vi "Goalie.vi"(9 "IA Input":T3, 10 "Robot":T1, 11 "command\nenum":T7) -> (2 "output cluster":T1)   [LabVIEW 2016]
uses:
  Core/AI Robot.ctl
  Functions Enum.ctl
  Command Enum.ctl
  Core/AI Input.ctl
  Core/AI Ball.ctl
  Core/Field Size.ctl
  Core/AI Judge.ctl
  <vilib>/Analysis/_algsub.llb/Real Vector Norm.vi
  <vilib>/Analysis/NI_AALPro.lvlib
panel:
  in  "min dist to kick 2":dbl=195.0 format="%#_13g"
  in  "attck contra?":dbl
  in  "min dist to kick":dbl=195.0 format="%#_13g"
  in  "T":dbl[](array[numeric])
  in  "Vel min":dbl=10.0 format="%#_13g"
  in  "Attacker Distance":dbl=200.0
  out "Closest Robot":T1
  out "Max Dist":dbl=999999999.0 format="%#_13g"
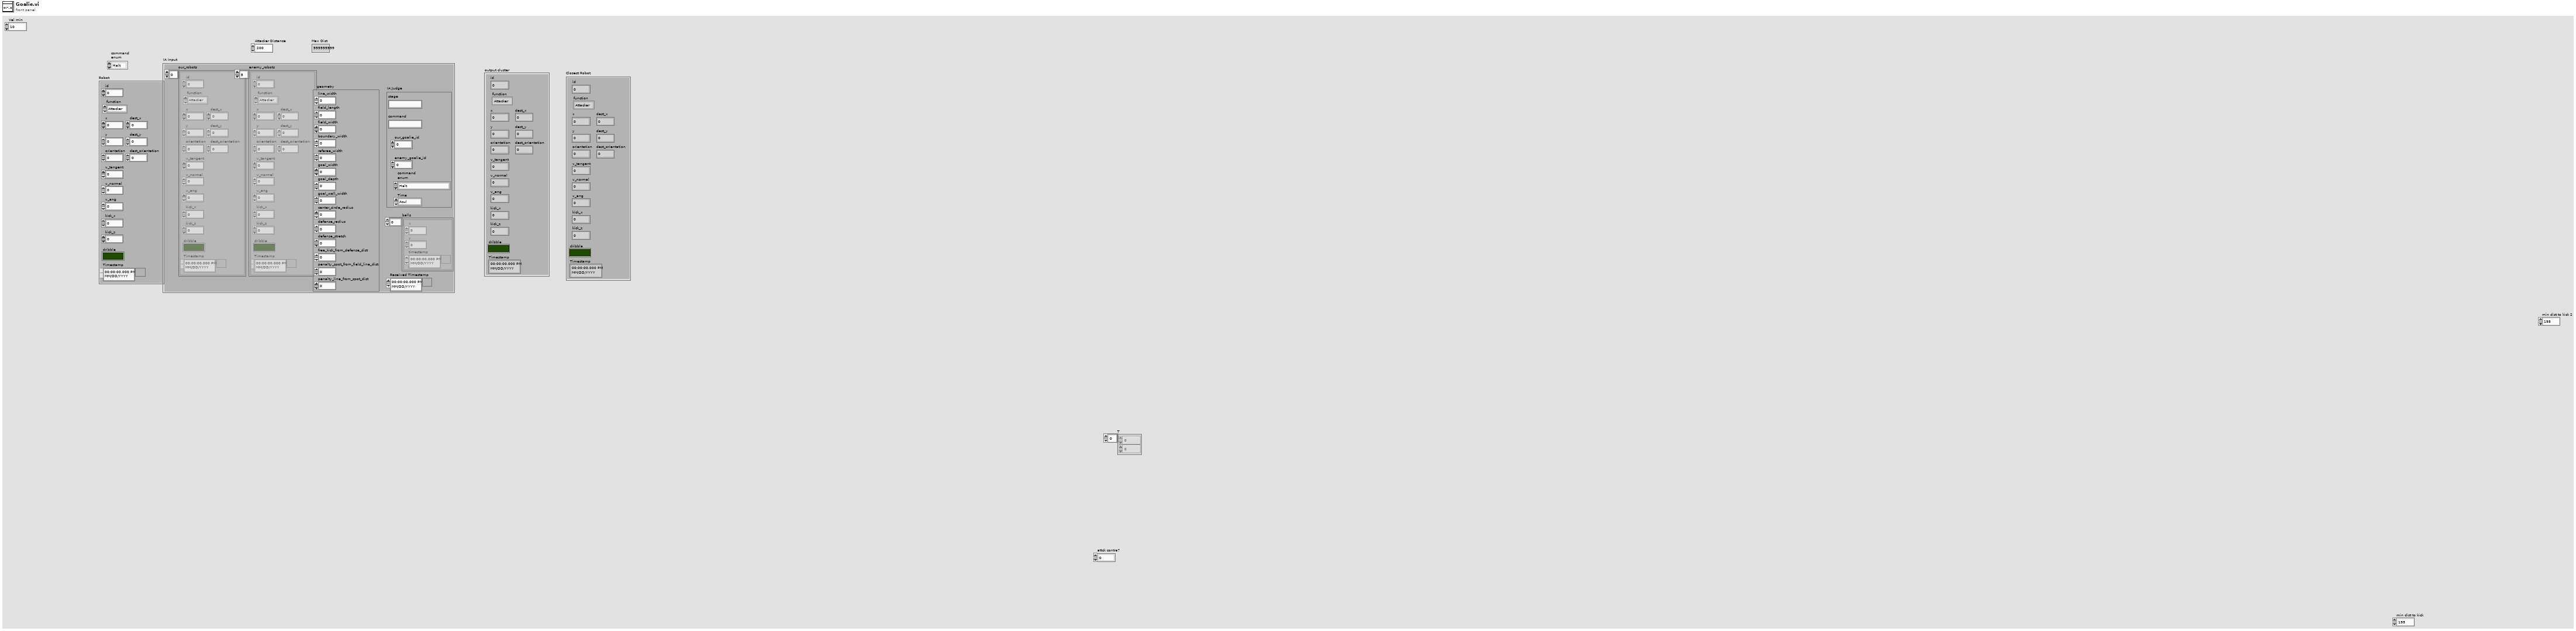
[diagram p1: front panel]
types:
  T1 = typedef "AI Robot.ctl" = cluster{"id":u32, "function":T2, "x":dbl, "y":dbl, "orientation":dbl, "v_tangent":dbl, "v_normal":dbl, "v_ang":dbl, "kick_x":dbl, "kick_z":dbl, "dribble":bool, "Timestamp":timestamp, "dest_x":dbl, "dest_y":dbl, "dest_orientation":dbl}
  T2 = typedef "Functions Enum.ctl" = enum16{"Attacker", "Goalie", "Defender", "Goto 0", "Dummy", "ZigZag"}
  T3 = typedef "AI Input.ctl" = cluster{"our_robots":T1[], "enemy_robots":T1[], "balls":T4[], "geometry":T5, "IA Judge":T6, "Received Timestamp":timestamp}
  T4 = typedef "AI Ball.ctl" = cluster{"x":dbl, "y":dbl, "timestamp":timestamp}
  T5 = typedef "Field Size.ctl" = cluster{"line_width":u32, "field_length":u32, "field_width":u32, "boundary_width":u32, "referee_width":u32, "goal_width":u32, "goal_depth":u32, "goal_wall_width":u32, "center_circle_radius":u32, "defense_radius":u32, "defense_stretch":u32, "free_kick_from_defense_dist":u32, "penalty_spot_from_field_line_dist":u32, "penalty_line_from_spot_dist":u32}
  T6 = typedef "AI Judge.ctl" = cluster{"stage":string, "command":string, "our_goalie_id":dbl, "enemy_goalie_id":dbl, "command\nenum":T7, "Time":enum16{"Azul", "Amarelo"}}
  T7 = typedef "Command Enum.ctl" = enum16{"Halt", "Stop", "Force Start", "PKA Normal Start", "Prepare Kickoff Ally", "PKE Normal Start", "Prepare Kickoff Enemy", "Prepare Penalty Ally", "PPA Normal Start", "Prepare Penalty Enemy", "PPE Normal Start", "Direct Free Enemy", "Direct Free Ally", "Indirect Free Enemy", "Indirect Free Ally", "Timeout Enemy", "Timeout Ally", "Goal Enemy", "Goal Ally", "Ball Placement Enemy", "Ball Placement Ally", "None"}
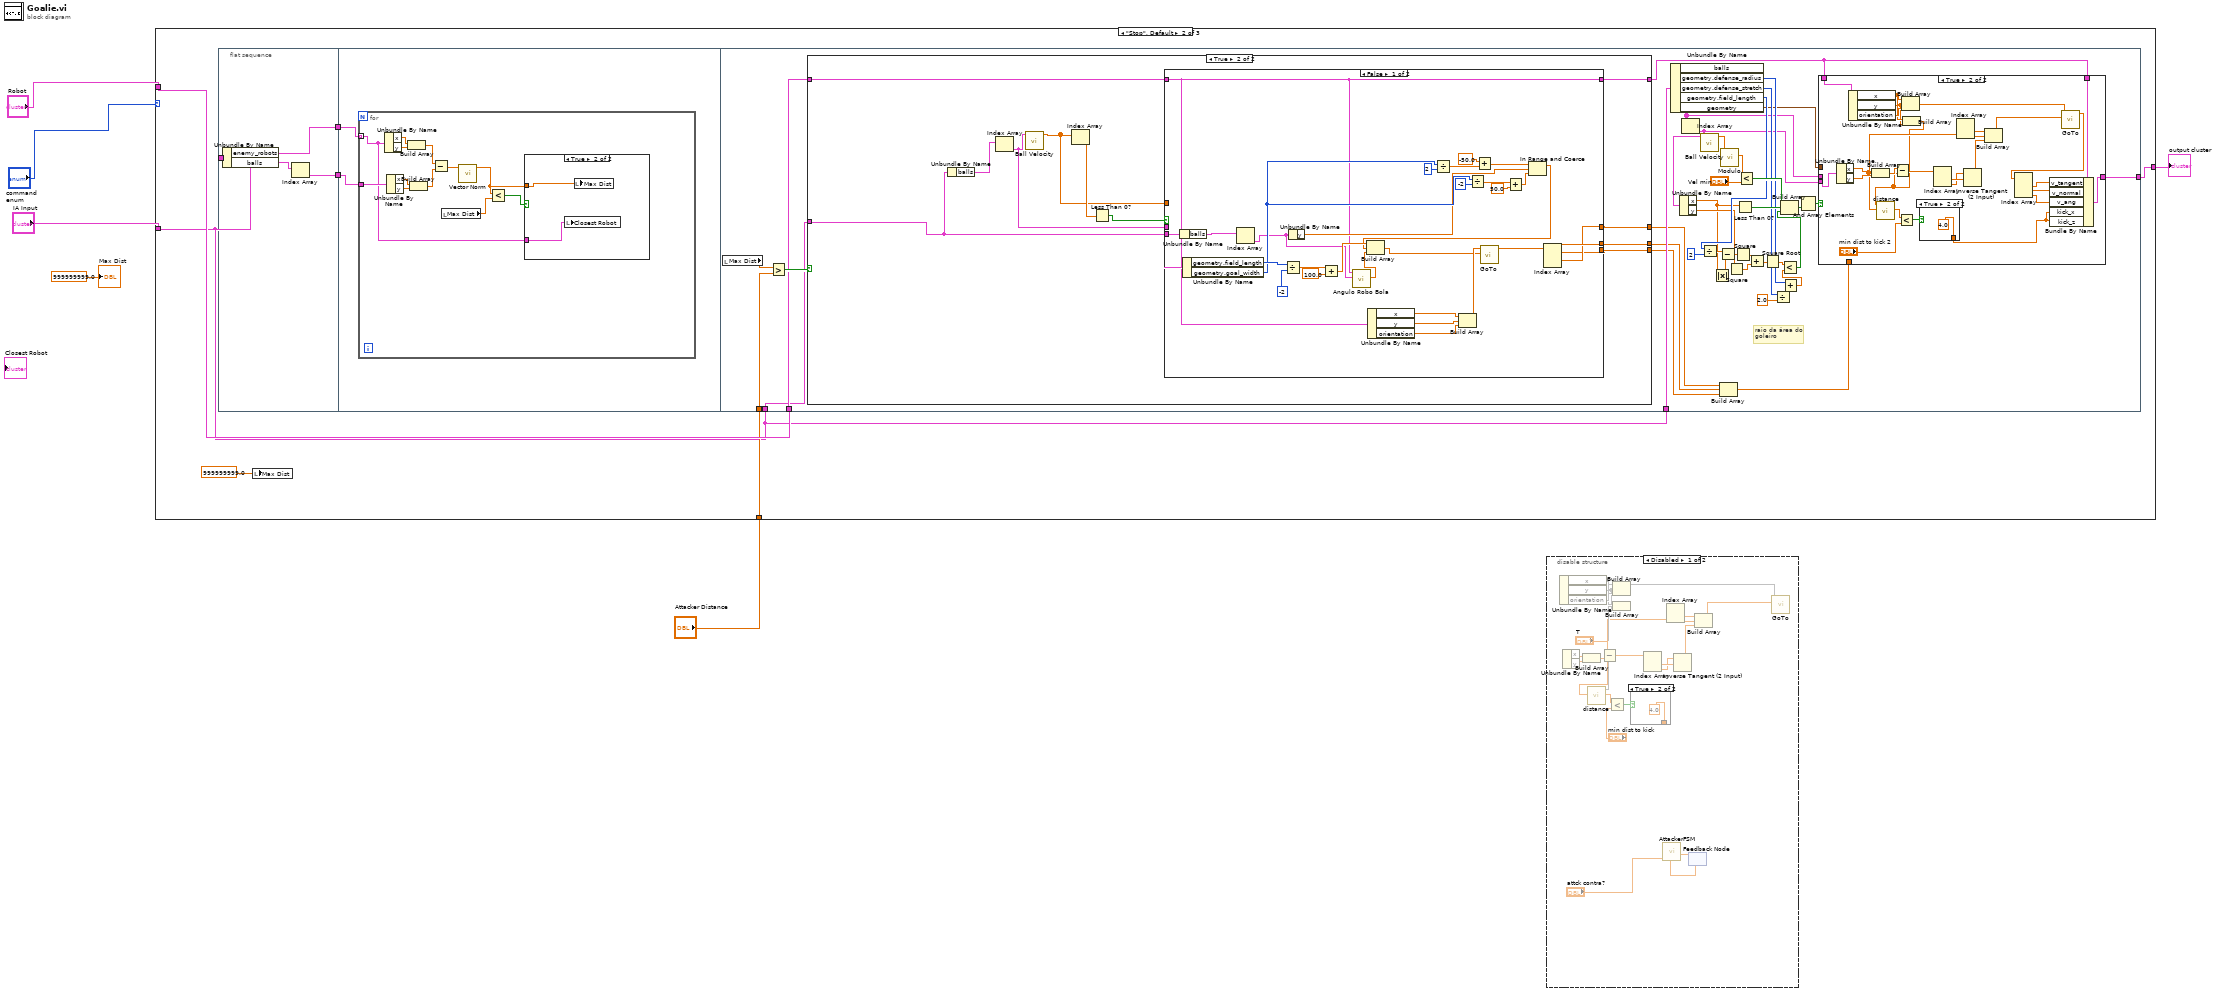
[diagram p0: block diagram]
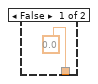
[diagram p2: hidden frame]
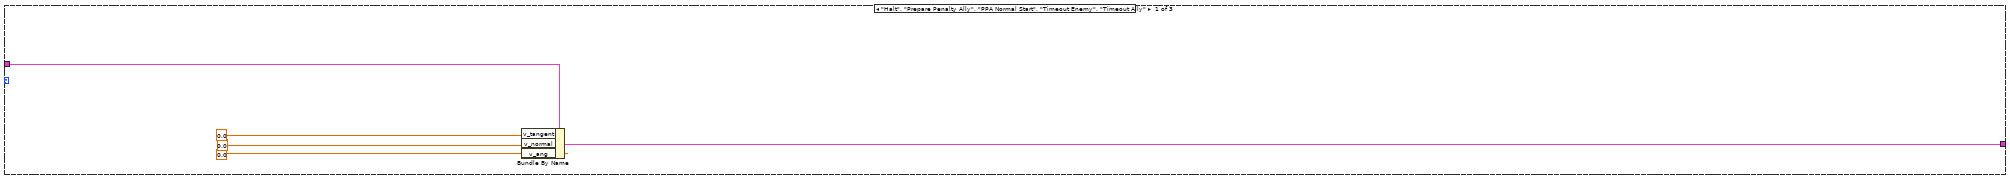
[diagram p4: hidden frame]
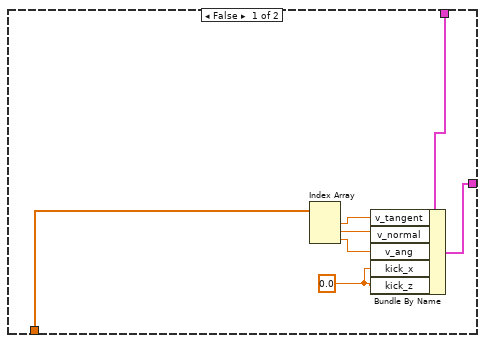
[diagram p6: hidden frame]
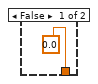
[diagram p7: hidden frame]
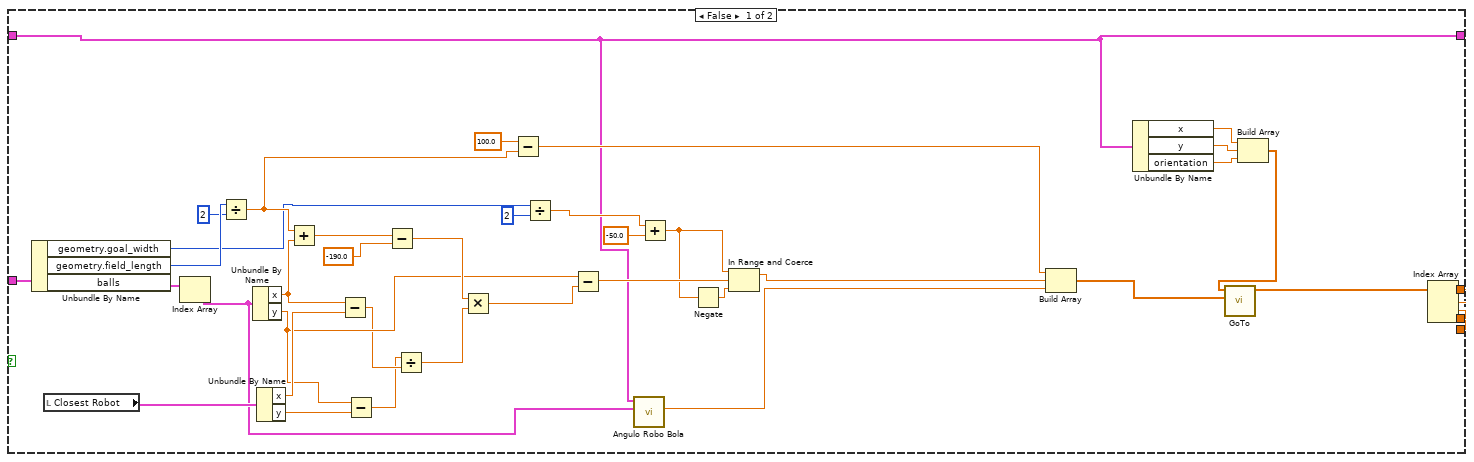
[diagram p8: hidden frame]
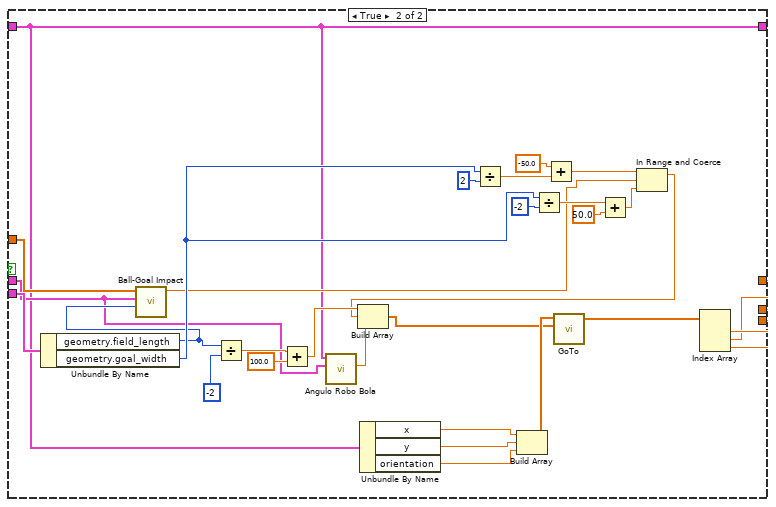
[diagram p9: hidden frame]
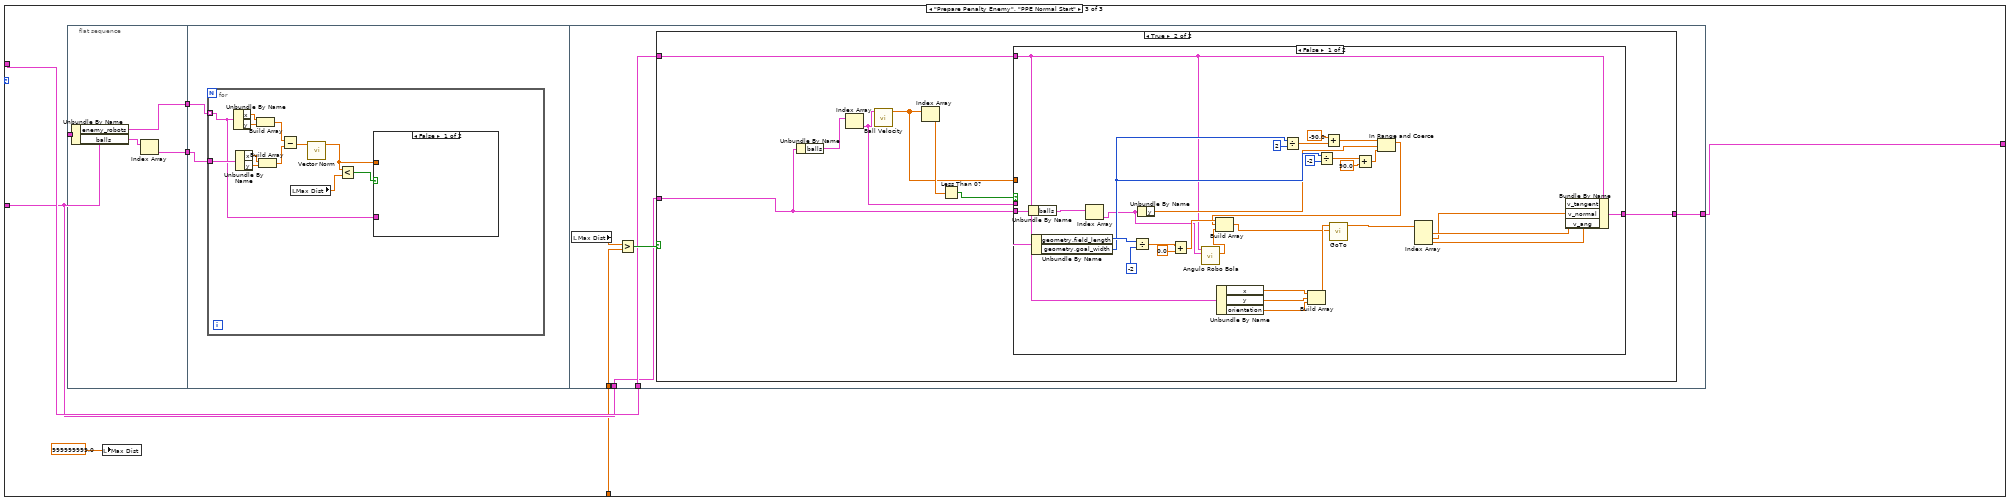
[diagram p10: hidden frame]
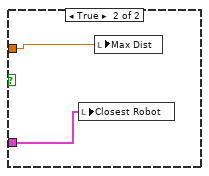
[diagram p11: hidden frame]
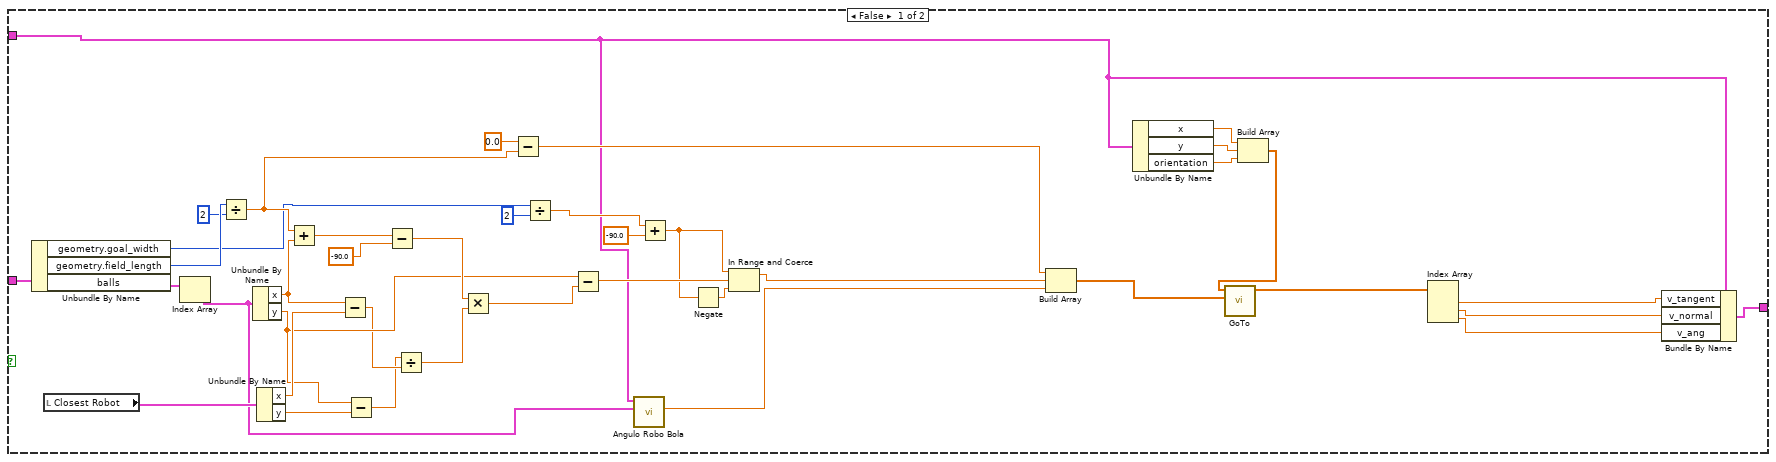
[diagram p12: hidden frame]
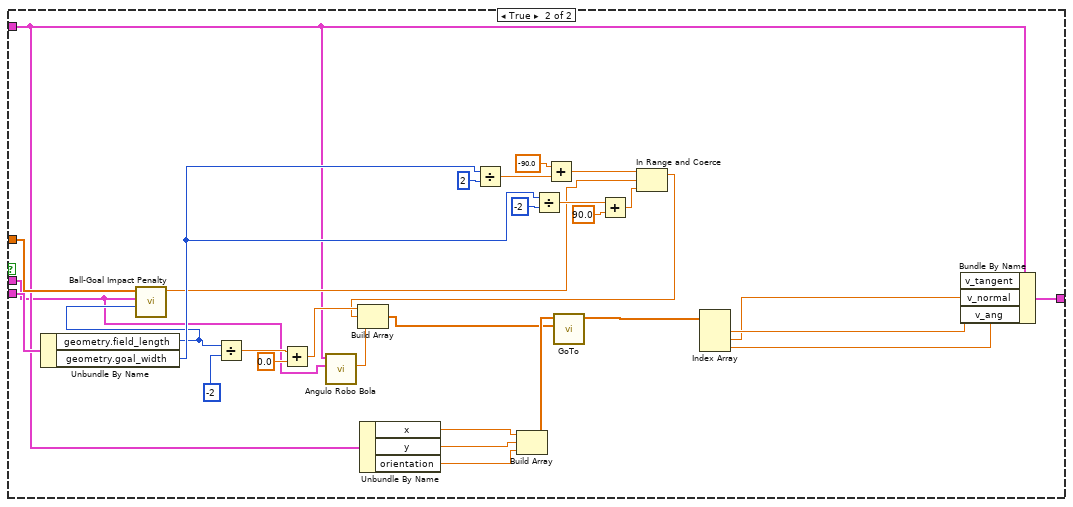
[diagram p13: hidden frame]
diagram:
  n1 = case shown="\"Stop\", Default" "command\nenum" {
    tunnel: "Robot" -> [w11 w16 w228]
    tunnel: [w7 w12 w226] -> w3
    tunnel: "IA Input" -> [_ w13 w227]
    tunnel: "Attacker Distance" -> [_ w15 w225]
    frame "Halt", "Prepare Penalty Ally", "PPA Normal Start", "Timeout Enemy", "Timeout Ally" {
      n2 = Bundle By Name(cluster=w11, "v_tangent"=0.0 ("v_x"), "v_normal"=0.0 ("v_y"), "v_ang"=0.0) -> (w7:T1)
    }
    frame "Stop", Default {
      n3 = flat-sequence {
        tunnel: w13 -> [w22]
        tunnel: [w21] -> w18
        tunnel: [w19] -> w17
        tunnel: w18 -> [w24]
        tunnel: w17 -> [w23]
        tunnel: w16 -> [w75]
        tunnel: w13 -> [w74]
        tunnel: w15 -> [w73]
        tunnel: w13 -> [w72]
        tunnel: [w41] -> w12
        frame #0 {
          n4 = Unbundle By Name(w22) -> ("enemy_robots"=w21:T1[], "balls"=w20:T4[])
          n5 = Index Array(array=w20) -> (element=w19:T4)  [unwired: 1 in]
        }
        frame #1 {
          n6 = for {
            tunnel: w24 -> [w26] mode=indexing
            tunnel: w23 -> [w36]
            n7 = Unbundle By Name(w26) -> ("x"=w35:dbl, "y"=w34:dbl)
            n8 = Unbundle By Name(w36) -> ("x"=w33:dbl, "y"=w32:dbl)
            n9 = Build Array(w35, w34) -> (w31:dbl[])
            n10 = Build Array(w33, w32) -> (w30:dbl[])
            n11 = Subtract(x=w31, y=w30) -> (x-y=w29:dbl[])
            n12 = local read "Max Dist"() -> (w28:dbl)
            n13 = call-poly <vilib>:"Vector Norm.vi"("Input Vector"=w29) -> ("norm"=w25:dbl)  [unwired: 9 in, 1 out]
            n14 = Less?(x=w25, y=w28) -> (x < y?=w27:bool)
            n15 = case shown="True" w27 {
              tunnel: w26 -> [_ w38]
              tunnel: w25 -> [_ w37]
              frame False {
              }
              frame True {
                n16 = local write "Closest Robot"(w38) -> ()
                n17 = local write "Max Dist"(w37) -> ()
              }
            }
          }
        }
        frame #2 {
          # "raio da área do \ngoleiro"
          n18 = local read "Max Dist"() -> (w76:dbl)
          n19 = Greater?(x=w76, y=w73) -> (0:w77:bool)
          n20 = case shown="True" w77 {
            tunnel: w75 -> [w114 w163]
            tunnel: w74 -> [w152 w162]
            tunnel: [w117 w156] -> w68
            tunnel: [w116 w155] -> w66
            tunnel: [w115 w154] -> w69
            tunnel: [w114 w153] -> w40
            frame False {
              n21 = Unbundle By Name(w152) -> ("geometry.goal_width"=w126:u32, "geometry.field_length"=w148:u32, "balls"=w151:T4[])
              n22 = local read "Closest Robot"() -> (w150:T1)
              n23 = Index Array(array=w151) -> (element=w119:T4)  [unwired: 1 in]
              n24 = Divide(x=w148, y=u32 2) -> (x/y=w137:dbl)
              n25 = Unbundle By Name(w119) -> ("x"=w146:dbl, "y"=w140:dbl)
              n26 = Unbundle By Name(w150) -> ("x"=w149:dbl, "y"=w139:dbl)
              n27 = Add(x=w137, y=w146) -> (x+y=w145:dbl)
              n28 = Subtract(x=w146, y=w149) -> (x-y=w129:dbl)
              n29 = Subtract(x=w140, y=w139) -> (x-y=w128:dbl)
              n30 = Subtract(x=w145, y=-190.0) -> (x-y=w143:dbl)
              n31 = Divide(x=w128, y=w129) -> (x/y=w142:dbl)
              n32 = Multiply(x=w143, y=w142) -> (x*y=w141:dbl)
              n33 = Subtract(x=100.0, y=w137) -> (x-y=w136:dbl)
              n34 = Divide(x=w126, y=u32 2) -> (x/y=w124:dbl)
              n35 = Subtract(x=w140, y=w141) -> (x-y=w127:dbl)
              n36 = call "Angulo Robo Bola.vi"("Ball"=w119, "Robot"=w114) -> ("Angulo"=w118:dbl)  [unwired: 9 in]
              n37 = Add(x=w124, y=-50.0) -> (x+y=w121:dbl)
              n38 = Negate(x=w121) -> (-x=w122:dbl)
              n39 = In Range and Coerce(upper limit=w121, x=w127, lower limit=w122) -> (coerced(x)=w120:dbl)  [unwired: 1 out]
              n40 = Build Array(w136, w120, w118) -> (w135:dbl[])
              n41 = Unbundle By Name(w114) -> ("x"=w134:dbl, "y"=w133:dbl, "orientation"=w132:dbl)
              n42 = Build Array(w134, w133, w132) -> (w131:dbl[])
              n43 = call "GoTo.vi"("Target"=w135, "Position"=w131) -> ("Output\nVelocity"=w130:dbl[])  [unwired: 8 in, 1 out]
              n44 = Index Array(array=w130) -> (element #1=w117:dbl, element #2=w116:dbl, element #3=w115:dbl)  [unwired: 3 in]
            }
            frame True {
              n45 = Unbundle By Name(w162) -> ("balls"=w161:T4[])
              n46 = Index Array(array=w161) -> (element=w157:T4)  [unwired: 1 in]
              n47 = call "Ball Velocity.vi"("Ball"=w157) -> ("Velocity"=w158:dbl[])  [unwired: 10 in]
              n48 = Index Array(array=w158) -> (element=w160:dbl)  [unwired: 1 in]
              n49 = Less Than 0?(x=w160) -> (x < 0?=w159:bool)
              n50 = case shown="False" w159 {
                tunnel: w162 -> [w189 w219]
                tunnel: w163 -> [w167 w194]
                tunnel: w158 -> [_ w201]
                tunnel: w157 -> [_ w199]
                tunnel: [w166 w197] -> w156
                tunnel: [w165 w196] -> w155
                tunnel: [w164 w195] -> w154
                tunnel: [w167 w194] -> w153
                frame False {
                  n51 = Unbundle By Name(w189) -> ("balls"=w188:T4[])
                  n52 = Unbundle By Name(w189) -> ("geometry.field_length"=w187:u32, "geometry.goal_width"=w180:u32)
                  n53 = Index Array(array=w188) -> (element=w169:T4)  [unwired: 1 in]
                  n54 = Divide(x=w187, y=-2) -> (x/y=w186:dbl)
                  n55 = Unbundle By Name(w169) -> ("y"=w176:dbl)
                  n56 = Add(x=w186, y=100.0) -> (x+y=w184:dbl)
                  n57 = call "Angulo Robo Bola.vi"("Ball"=w169, "Robot"=w167) -> ("Angulo"=w168:dbl)  [unwired: 9 in]
                  n58 = Unbundle By Name(w167) -> ("x"=w191:dbl, "y"=w193:dbl, "orientation"=w192:dbl)
                  n59 = Divide(x=w180, y=2) -> (x/y=w173:dbl)
                  n60 = Build Array(w191, w193, w192) -> (w183:dbl[])
                  n61 = Divide(x=w180, y=-2) -> (x/y=w175:dbl)
                  n62 = Add(x=-50.0, y=w173) -> (x+y=w171:dbl)
                  n63 = Add(x=w175, y=50.0) -> (x+y=w170:dbl)
                  n64 = In Range and Coerce(upper limit=w171, x=w176, lower limit=w170) -> (coerced(x)=w177:dbl)  [unwired: 1 out]
                  n65 = Build Array(w184, w177, w168) -> (w182:dbl[])
                  n66 = call "GoTo.vi"("Target"=w182, "Position"=w183) -> ("Output\nVelocity"=w181:dbl[])  [unwired: 8 in, 1 out]
                  n67 = Index Array(array=w181) -> (element #1=w166:dbl, element #2=w165:dbl, element #3=w164:dbl)  [unwired: 3 in]
                }
                frame True {
                  n68 = Unbundle By Name(w219) -> ("geometry.field_length"=w202:u32, "geometry.goal_width"=w212:u32)
                  n69 = call "Ball-Goal Impact.vi"("Field Length"=w202, "Ball"=w199, "Ball Velocity"=w201) -> ("Y Collision"=w200:dbl)  [unwired: 8 in]
                  n70 = Divide(x=w202, y=-2) -> (x/y=w218:dbl)
                  n71 = Add(x=w218, y=100.0) -> (x+y=w216:dbl)
                  n72 = call "Angulo Robo Bola.vi"("Ball"=w199, "Robot"=w194) -> ("Angulo"=w198:dbl)  [unwired: 9 in]
                  n73 = Unbundle By Name(w194) -> ("x"=w221:dbl, "y"=w223:dbl, "orientation"=w222:dbl)
                  n74 = Divide(x=w212, y=2) -> (x/y=w206:dbl)
                  n75 = Build Array(w221, w223, w222) -> (w215:dbl[])
                  n76 = Divide(x=w212, y=-2) -> (x/y=w208:dbl)
                  n77 = Add(x=-50.0, y=w206) -> (x+y=w204:dbl)
                  n78 = Add(x=w208, y=50.0) -> (x+y=w203:dbl)
                  n79 = In Range and Coerce(upper limit=w204, x=w200, lower limit=w203) -> (coerced(x)=w209:dbl)  [unwired: 1 out]
                  n80 = Build Array(w216, w209, w198) -> (w214:dbl[])
                  n81 = call "GoTo.vi"("Target"=w214, "Position"=w215) -> ("Output\nVelocity"=w213:dbl[])  [unwired: 8 in, 1 out]
                  n82 = Index Array(array=w213) -> (element #1=w197:dbl, element #2=w196:dbl, element #3=w195:dbl)  [unwired: 3 in]
                }
              }
            }
          }
          n83 = Unbundle By Name(w72) -> ("balls"=w43:T4[], "geometry.defense_radius"=w54:u32, "geometry.defense_stretch"=w56:u32, "geometry.field_length"=w50:u32, "geometry"=w42:T5)
          n84 = Index Array(array=w43) -> (element=w39:T4)  [unwired: 1 in]
          n85 = Unbundle By Name(w39) -> ("x"=w45:dbl, "y"=w48:dbl)
          n86 = call "Ball Velocity.vi"("Ball"=w39) -> ("Velocity"=w71:dbl[])  [unwired: 10 in]
          n87 = Divide(x=w50, y=u32 2) -> (x/y=w51:dbl)
          n88 = Absolute Value(x=w45) -> (abs(x)=w44:dbl)
          n89 = Subtract(x=w51, y=w44) -> (x-y=w60:dbl)
          n90 = Build Array(w68, w66, w69) -> (w67:dbl[])
          n91 = call "Modulo.vi"("2D vector"=w71) -> ("Modulo"=w70:dbl)  [unwired: 10 in]
          n92 = Square(x=w48) -> (x^2=w59:dbl)
          n93 = Square(x=w60) -> (x^2=w58:dbl)
          n94 = Less Than 0?(x=w45) -> (x < 0?=w61:bool)
          n95 = Less?(x=w70, y="Vel min") -> (x < y?=w63:bool)
          n96 = Add(x=w58, y=w59) -> (x+y=w46:dbl)
          n97 = Square Root(x=w46) -> (sqrt(x)=w47:dbl)
          n98 = Divide(x=w56, y=2.0) -> (x/y=w57:dbl)
          n99 = Add(x=w54, y=w57) -> (x+y=w53:dbl)
          n100 = Less?(x=w47, y=w53) -> (x < y?=w52:bool)
          n101 = Build Array(w63, w61, w52) -> (w65:bool[])
          n102 = And Array Elements(Boolean array=w65) -> (logical AND=w64:bool)
          n103 = case shown="True" w64 {
            tunnel: w43 -> [_ _]
            tunnel: w40 -> [_ w95]
            tunnel: w67 -> [w79 _]
            tunnel: w42 -> [_ _]
            tunnel: [w81 w89] -> w41
            tunnel: w40 -> [w80 w90]
            tunnel: w39 -> [_ w87]
            frame False {
              w78 = 0.0
              n104 = Index Array(array=w79) -> (element #1=w84:dbl, element #2=w83:dbl, element #3=w82:dbl)  [unwired: 3 in]
              n105 = Bundle By Name(cluster=w80, "v_tangent"=w84, "v_normal"=w83, "v_ang"=w82, "kick_x"=w78, "kick_z"=w78) -> (w81:T1)
            }
            frame True {
              n106 = Unbundle By Name(w87) -> ("x"=w105:dbl, "y"=w104:dbl)
              n107 = Unbundle By Name(w95) -> ("x"=w110:dbl, "y"=w109:dbl, "orientation"=w111:dbl)
              n108 = Build Array(w105, w104) -> (w86:dbl[])
              n109 = Build Array(w110, w109, w111) -> (w108:dbl[])
              n110 = Build Array(w110, w109) -> (w85:dbl[])
              n111 = call "distance.vi"("target pos"=w86, "obj pos"=w85) -> ("sqrt(x)"=w96:dbl)  [unwired: 9 in]
              n112 = Subtract(x=w86, y=w85) -> (x-y=w103:dbl[])
              n113 = Less?(x=w96, y="min dist to kick 2") -> (x < y?=w98:bool)
              n114 = case shown="True" w98 {
                tunnel: [0.0 4.0] -> w88
                frame False {
                }
                frame True {
                }
              }
              n115 = Index Array(array=w103) -> (element #1=w107:dbl, element #2=w106:dbl)  [unwired: 2 in]
              n116 = Index Array(array=w86) -> (element #1=w100:dbl, element #2=w99:dbl)  [unwired: 2 in]
              n117 = Inverse Tangent (2 Input)(1:w107, 2:w106) -> (0:w101:dbl)
              n118 = Build Array(w100, w99, w101) -> (w102:dbl[])
              n119 = call "GoTo.vi"("Target"=w102, "Position"=w108) -> ("Output\nVelocity"=w91:dbl[])  [unwired: 8 in, 1 out]
              n120 = Index Array(array=w91) -> (element #1=w92:dbl, element #2=w93:dbl, element #3=w94:dbl)  [unwired: 3 in]
              n121 = Bundle By Name(cluster=w90, "v_tangent"=w92, "v_normal"=w93, "v_ang"=w94, "kick_x"=w88, "kick_z"=w88) -> (w89:T1)
            }
          }
        }
      }
      n122 = local write "Max Dist"(999999999.0 ("Max Dist")) -> ()
    }
    frame "Prepare Penalty Enemy", "PPE Normal Start" {
      n123 = flat-sequence {
        tunnel: w227 -> [w234]
        tunnel: [w233] -> w230
        tunnel: [w231] -> w229
        tunnel: w230 -> [w236]
        tunnel: w229 -> [w235]
        tunnel: w228 -> [w254]
        tunnel: w227 -> [w253]
        tunnel: [w252] -> w226
        tunnel: w225 -> [w251]
        frame #0 {
          n124 = Unbundle By Name(w234) -> ("enemy_robots"=w233:T1[], "balls"=w232:T4[])
          n125 = Index Array(array=w232) -> (element=w231:T4)  [unwired: 1 in]
        }
        frame #1 {
          n126 = for {
            tunnel: w236 -> [w238] mode=indexing
            tunnel: w235 -> [w248]
            n127 = Unbundle By Name(w238) -> ("x"=w247:dbl, "y"=w246:dbl)
            n128 = Unbundle By Name(w248) -> ("x"=w245:dbl, "y"=w244:dbl)
            n129 = Build Array(w247, w246) -> (w243:dbl[])
            n130 = Build Array(w245, w244) -> (w242:dbl[])
            n131 = Subtract(x=w243, y=w242) -> (x-y=w241:dbl[])
            n132 = local read "Max Dist"() -> (w240:dbl)
            n133 = call-poly <vilib>:"Vector Norm.vi"("Input Vector"=w241) -> ("norm"=w237:dbl)  [unwired: 9 in, 1 out]
            n134 = Less?(x=w237, y=w240) -> (x < y?=w239:bool)
            n135 = case shown="False" w239 {
              tunnel: w238 -> [_ w250]
              tunnel: w237 -> [_ w249]
              frame False {
              }
              frame True {
                n136 = local write "Closest Robot"(w250) -> ()
                n137 = local write "Max Dist"(w249) -> ()
              }
            }
          }
        }
        frame #2 {
          n138 = local read "Max Dist"() -> (w255:dbl)
          n139 = Greater?(x=w255, y=w251) -> (0:w256:bool)
          n140 = case shown="True" w256 {
            tunnel: w254 -> [w259 w304]
            tunnel: [w270 w303] -> w252
            tunnel: w253 -> [w296 w302]
            frame False {
              n141 = Unbundle By Name(w296) -> ("geometry.goal_width"=w266:u32, "geometry.field_length"=w292:u32, "balls"=w295:T4[])
              n142 = local read "Closest Robot"() -> (w294:T1)
              n143 = Index Array(array=w295) -> (element=w258:T4)  [unwired: 1 in]
              n144 = Divide(x=w292, y=u32 2) -> (x/y=w281:dbl)
              n145 = Unbundle By Name(w258) -> ("x"=w290:dbl, "y"=w284:dbl)
              n146 = Unbundle By Name(w294) -> ("x"=w293:dbl, "y"=w283:dbl)
              n147 = Add(x=w281, y=w290) -> (x+y=w289:dbl)
              n148 = Subtract(x=w290, y=w293) -> (x-y=w269:dbl)
              n149 = Subtract(x=w284, y=w283) -> (x-y=w268:dbl)
              n150 = Subtract(x=w289, y=-90.0) -> (x-y=w287:dbl)
              n151 = Divide(x=w268, y=w269) -> (x/y=w286:dbl)
              n152 = Multiply(x=w287, y=w286) -> (x*y=w285:dbl)
              n153 = Subtract(x=0.0, y=w281) -> (x-y=w280:dbl)
              n154 = Divide(x=w266, y=u32 2) -> (x/y=w264:dbl)
              n155 = Subtract(x=w284, y=w285) -> (x-y=w267:dbl)
              n156 = call "Angulo Robo Bola.vi"("Ball"=w258, "Robot"=w259) -> ("Angulo"=w257:dbl)  [unwired: 9 in]
              n157 = Add(x=w264, y=-90.0) -> (x+y=w261:dbl)
              n158 = Negate(x=w261) -> (-x=w262:dbl)
              n159 = In Range and Coerce(upper limit=w261, x=w267, lower limit=w262) -> (coerced(x)=w260:dbl)  [unwired: 1 out]
              n160 = Build Array(w280, w260, w257) -> (w279:dbl[])
              n161 = Unbundle By Name(w259) -> ("x"=w278:dbl, "y"=w277:dbl, "orientation"=w276:dbl)
              n162 = Build Array(w278, w277, w276) -> (w275:dbl[])
              n163 = call "GoTo.vi"("Target"=w279, "Position"=w275) -> ("Output\nVelocity"=w274:dbl[])  [unwired: 8 in, 1 out]
              n164 = Index Array(array=w274) -> (element #1=w273:dbl, element #2=w272:dbl, element #3=w271:dbl)  [unwired: 3 in]
              n165 = Bundle By Name(cluster=w259, "v_tangent"=w273, "v_normal"=w272, "v_ang"=w271) -> (w270:T1)
            }
            frame True {
              n166 = Unbundle By Name(w302) -> ("balls"=w301:T4[])
              n167 = Index Array(array=w301) -> (element=w297:T4)  [unwired: 1 in]
              n168 = call "Ball Velocity.vi"("Ball"=w297) -> ("Velocity"=w298:dbl[])  [unwired: 10 in]
              n169 = Index Array(array=w298) -> (element=w300:dbl)  [unwired: 1 in]
              n170 = Less Than 0?(x=w300) -> (x < 0?=w299:bool)
              n171 = case shown="False" w299 {
                tunnel: w302 -> [w331 w362]
                tunnel: w304 -> [w307 w338]
                tunnel: [w319 w352] -> w303
                tunnel: w298 -> [_ w340]
                tunnel: w297 -> [_ w337]
                frame False {
                  n172 = Unbundle By Name(w331) -> ("balls"=w330:T4[])
                  n173 = Unbundle By Name(w331) -> ("geometry.field_length"=w329:u32, "geometry.goal_width"=w318:u32)
                  n174 = Index Array(array=w330) -> (element=w306:T4)  [unwired: 1 in]
                  n175 = Divide(x=w329, y=-2) -> (x/y=w328:dbl)
                  n176 = Unbundle By Name(w306) -> ("y"=w314:dbl)
                  n177 = Add(x=w328, y=0.0) -> (x+y=w326:dbl)
                  n178 = call "Angulo Robo Bola.vi"("Ball"=w306, "Robot"=w307) -> ("Angulo"=w305:dbl)  [unwired: 9 in]
                  n179 = Unbundle By Name(w307) -> ("x"=w333:dbl, "y"=w335:dbl, "orientation"=w334:dbl)
                  n180 = Divide(x=w318, y=2) -> (x/y=w311:dbl)
                  n181 = Build Array(w333, w335, w334) -> (w325:dbl[])
                  n182 = Divide(x=w318, y=-2) -> (x/y=w313:dbl)
                  n183 = Add(x=-90.0, y=w311) -> (x+y=w309:dbl)
                  n184 = Add(x=w313, y=90.0) -> (x+y=w308:dbl)
                  n185 = In Range and Coerce(upper limit=w309, x=w314, lower limit=w308) -> (coerced(x)=w315:dbl)  [unwired: 1 out]
                  n186 = Build Array(w326, w315, w305) -> (w324:dbl[])
                  n187 = call "GoTo.vi"("Target"=w324, "Position"=w325) -> ("Output\nVelocity"=w323:dbl[])  [unwired: 8 in, 1 out]
                  n188 = Index Array(array=w323) -> (element #1=w322:dbl, element #2=w321:dbl, element #3=w320:dbl)  [unwired: 3 in]
                  n189 = Bundle By Name(cluster=w307, "v_tangent"=w322, "v_normal"=w321, "v_ang"=w320) -> (w319:T1)
                }
                frame True {
                  n190 = Unbundle By Name(w362) -> ("geometry.field_length"=w341:u32, "geometry.goal_width"=w351:u32)
                  n191 = call "Ball-Goal Impact Penalty.vi"("Field Length"=w341, "Ball"=w337, "Ball Velocity"=w340) -> ("Y Collision"=w339:dbl)  [unwired: 8 in]
                  n192 = Divide(x=w341, y=-2) -> (x/y=w361:dbl)
                  n193 = Add(x=w361, y=0.0) -> (x+y=w359:dbl)
                  n194 = call "Angulo Robo Bola.vi"("Ball"=w337, "Robot"=w338) -> ("Angulo"=w336:dbl)  [unwired: 9 in]
                  n195 = Unbundle By Name(w338) -> ("x"=w364:dbl, "y"=w366:dbl, "orientation"=w365:dbl)
                  n196 = Divide(x=w351, y=2) -> (x/y=w345:dbl)
                  n197 = Build Array(w364, w366, w365) -> (w358:dbl[])
                  n198 = Divide(x=w351, y=-2) -> (x/y=w347:dbl)
                  n199 = Add(x=-90.0, y=w345) -> (x+y=w343:dbl)
                  n200 = Add(x=w347, y=90.0) -> (x+y=w342:dbl)
                  n201 = In Range and Coerce(upper limit=w343, x=w339, lower limit=w342) -> (coerced(x)=w348:dbl)  [unwired: 1 out]
                  n202 = Build Array(w359, w348, w336) -> (w357:dbl[])
                  n203 = call "GoTo.vi"("Target"=w357, "Position"=w358) -> ("Output\nVelocity"=w356:dbl[])  [unwired: 8 in, 1 out]
                  n204 = Index Array(array=w356) -> (element #1=w355:dbl, element #2=w354:dbl, element #3=w353:dbl)  [unwired: 3 in]
                  n205 = Bundle By Name(cluster=w338, "v_tangent"=w355, "v_normal"=w354, "v_ang"=w353) -> (w352:T1)
                }
              }
            }
          }
        }
      }
      n206 = local write "Max Dist"(999999999.0 ("Max Dist")) -> ()
    }
  }
  "output cluster" <- w3
  n207 = disable-structure shown="Disabled" {
    frame Disabled {
      n208 = Unbundle By Name() -> (w395:T1, "x"=w393, "y"=w392, "orientation"=w394)
      n209 = Unbundle By Name() -> ("x"=w388:dbl, "y"=w387:dbl)  [unwired: 1 in]
      n210 = Build Array(w388, w387) -> (w375:dbl[])
      n211 = Subtract(x="T", y=w375) -> (x-y=w385:dbl[])
      n212 = Build Array(w393, w392, w394) -> (w391:void[])
      n213 = Build Array(w393, w392) -> (w376:void[])
      n214 = call "distance.vi"("target pos"=w375, "obj pos"=w376) -> ("sqrt(x)"=w374:dbl)  [unwired: 9 in]
      n215 = Less?(x=w374, y="min dist to kick") -> (x < y?=w379:bool)
      n216 = case shown="True" w379 {
        tunnel: [0.0 4.0] -> w377
        frame False {
        }
        frame True {
        }
      }
      n217 = Index Array(array=w385) -> (element #1=w390:dbl, element #2=w389:dbl)  [unwired: 2 in]
      n218 = Index Array(array=w375) -> (element #1=w382:dbl, element #2=w381:dbl)  [unwired: 2 in]
      n219 = Inverse Tangent (2 Input)(1:w390, 2:w389) -> (0:w383:dbl)
      n220 = feedback #1() -> (w370:dbl)  [unwired: 1 in]
      n221 = call "AttackerFSM.vi"("Current State"=w370, "attck contra?"="attck contra?") -> ("Next State"=w369:dbl, "Robot out"=w368:T1, "balls"=w371:T4[], "Field Size in"=w372:T5, "Robot in"=w373:T1)  [unwired: 5 in]
      n222 = feedback-in #1(w369) -> ()
      n223 = Build Array(w382, w381, w383) -> (w384:dbl[])
      n224 = call "GoTo.vi"("Target"=w384, "Position"=w391) -> ("Output\nVelocity"=w380:dbl[])  [unwired: 8 in, 1 out]
    }
    frame Enabled {
    }
  }
  "Max Dist" <- 999999999.0 ("Max Dist")
